vi "ep_Angle Convertor.vi"(0 "input angle":dbl, 1 "input unit (F: radian)":bool) -> (4 "angle in radians (0..2PI)":dbl, 6 "angle in radians (-PI..PI)":dbl, 8 "angle in degrees (0..360)":dbl, 10 "angle in degrees (-180..180)":dbl)   [LabVIEW 2011, in "NI_EP_Power Quality.lvlib"]
uses:
  <vilib>/addons/Electrical Power/PQ/NI_EP_Power Quality.lvlib
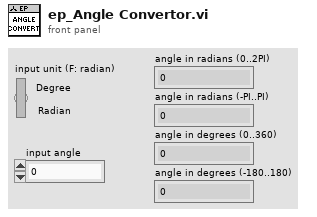
[diagram p1: front panel]
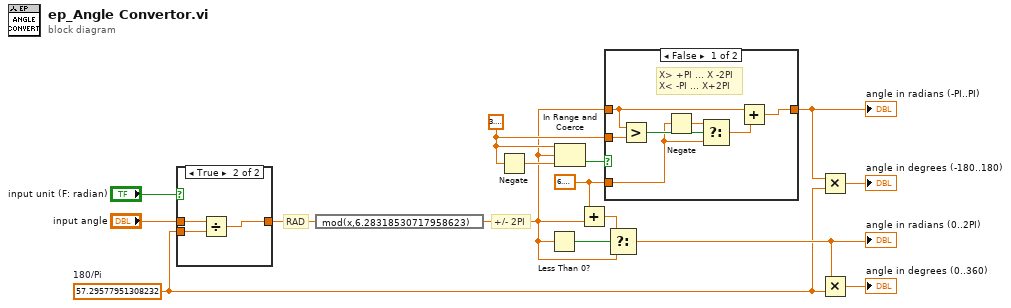
[diagram p0: block diagram]
diagram:
  w1 = 57.29577951308232  # 180/Pi
  w11 = 3.141592653589793
  w10 = 6.283185307179586
  # "RAD"
  # "+/- 2PI"
  n1 = case shown="True" "input unit (F: radian)" {
    tunnel: "input angle" -> [w16 w19]
    tunnel: w1 -> [_ w18]
    tunnel: [w16 w17] -> w7
    frame False {
    }
    frame True {
      n2 = Divide(x=w19, y=w18) -> (x/y=w17:dbl)
    }
  }
  n3 = expression code="mod(x,6.28318530717958623)"(w7) -> (w2:dbl)
  n4 = Negate(x=w11) -> (-x=w13:dbl)
  n5 = Less Than 0?(x=w2) -> (x < 0?=w15:bool)
  n6 = In Range and Coerce(upper limit=w11, x=w2, lower limit=w13) -> (In Range?=w12:bool)  [unwired: 1 out]
  n7 = Add(x=w10, y=w2) -> (x+y=w14:dbl)
  n8 = case shown="False" w12 {
    tunnel: w2 -> [w25 w27]
    tunnel: [w24 w27] -> w6
    tunnel: w11 -> [w26 _]
    tunnel: w10 -> [w21 _]
    frame False {
      # "X> +PI ... X -2PI\nX< -PI ... X+2PI"
      n9 = Greater?(x=w25, y=w26) -> (0:w23:bool)
      n10 = Negate(x=w21) -> (-x=w22:dbl)
      n11 = Select(t=w22, s=w23, f=w21) -> (s? t:f=w20:dbl)
      n12 = Add(x=w25, y=w20) -> (x+y=w24:dbl)
    }
    frame True {
    }
  }
  "angle in radians (-PI..PI)" <- w6
  n13 = Select(t=w14, s=w15, f=w2) -> (s? t:f=w3:dbl)
  "angle in radians (0..2PI)" <- w3
  n14 = Multiply(x=w6, y=w1) -> (x*y=→"angle in degrees (-180..180)":dbl)
  n15 = Multiply(x=w3, y=w1) -> (x*y=→"angle in degrees (0..360)":dbl)
